vi "Read and Add Instr CFGs.vi"(8 "error in":errorcluster, 10 "Instr CFGs":path[](array[path]), 11 "File Provider in":refnum<class "File Provider.lvclass">) -> (0 "error out":errorcluster, 3 "File Provider out":refnum<class "File Provider.lvclass">)   [LabVIEW 2024, in "File Provider.lvlib" / "File Provider.lvclass"]
uses:
  File Provider.lvclass
  File Provider.lvclass/File Provider.ctl
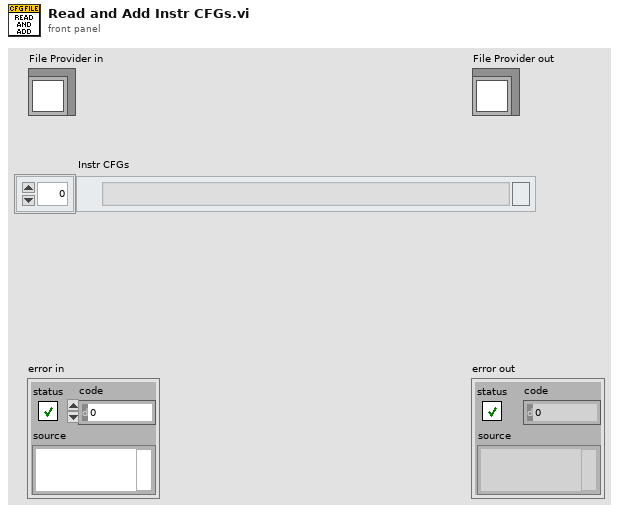
[diagram p1: front panel]
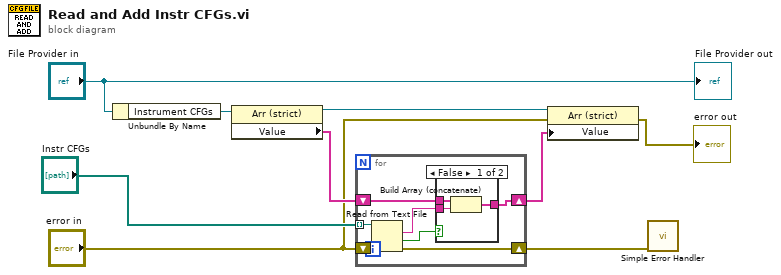
[diagram p0: block diagram]
diagram:
  n1 = Unbundle By Name("File Provider in") -> ("Instrument CFGs"=w6:refnum<vi>)
  n2 = property class="Arr (strict)"(reference=w6) -> (reference out=w4:refnum<vi>, "Value"=w5:string[])  [unwired: 1 in, 1 out]
  n3 = for {
    tunnel: "Instr CFGs" -> [w11] mode=indexing
    shift-right: [w16] -> w9
    shift-left: "error in" -> [w15]
    shift-right: [w10] -> w3
    shift-left: w5 -> [w13]
    n4 = Read from Text File(file (use dialog)=w11, error in=w15) -> (text=w12:string, cancelled=w14:bool, error out=w16:errorcluster)  [unwired: 2 in, 1 out]
    n5 = case shown="False" w14 {
      tunnel: w13 -> [w19 w20]
      tunnel: w12 -> [w18 _]
      tunnel: [w17 w20] -> w10
      frame False {
        n6 = Build Array (concatenate)(w19, w18) -> (w17:string[])
      }
      frame True {
      }
    }
  }
  n7 = property class="Arr (strict)"(reference=w4, error in="error in", "Value"=w3) -> (error out=→"error out":errorcluster)  [unwired: 1 out]
  n8 = call <vilib>:"Simple Error Handler.vi"("error in (no error)"=w9) -> ()  [unwired: 4 in, 5 out]
  "File Provider out" <- "File Provider in"
